vi "Sched select tube mask.vi"(9 "sched61-80mask":u32, 10 "sched31-60mask":u32, 11 "sched1-30mask":u32) -> (1 "Close":bool, 2 "Load":bool, 3 "selected sched":string)   [LabVIEW 2023]
uses:
  Sched select.ctl
panel:
  out "schd61-80array":bool[](array[boolean])
  out "schd31-60array":bool[](array[boolean])
  out "schd1-30array":bool[](array[boolean])
  in  "stop":bool
  in  "Schedules":T1
  out "SchedNames":string[](array[string])
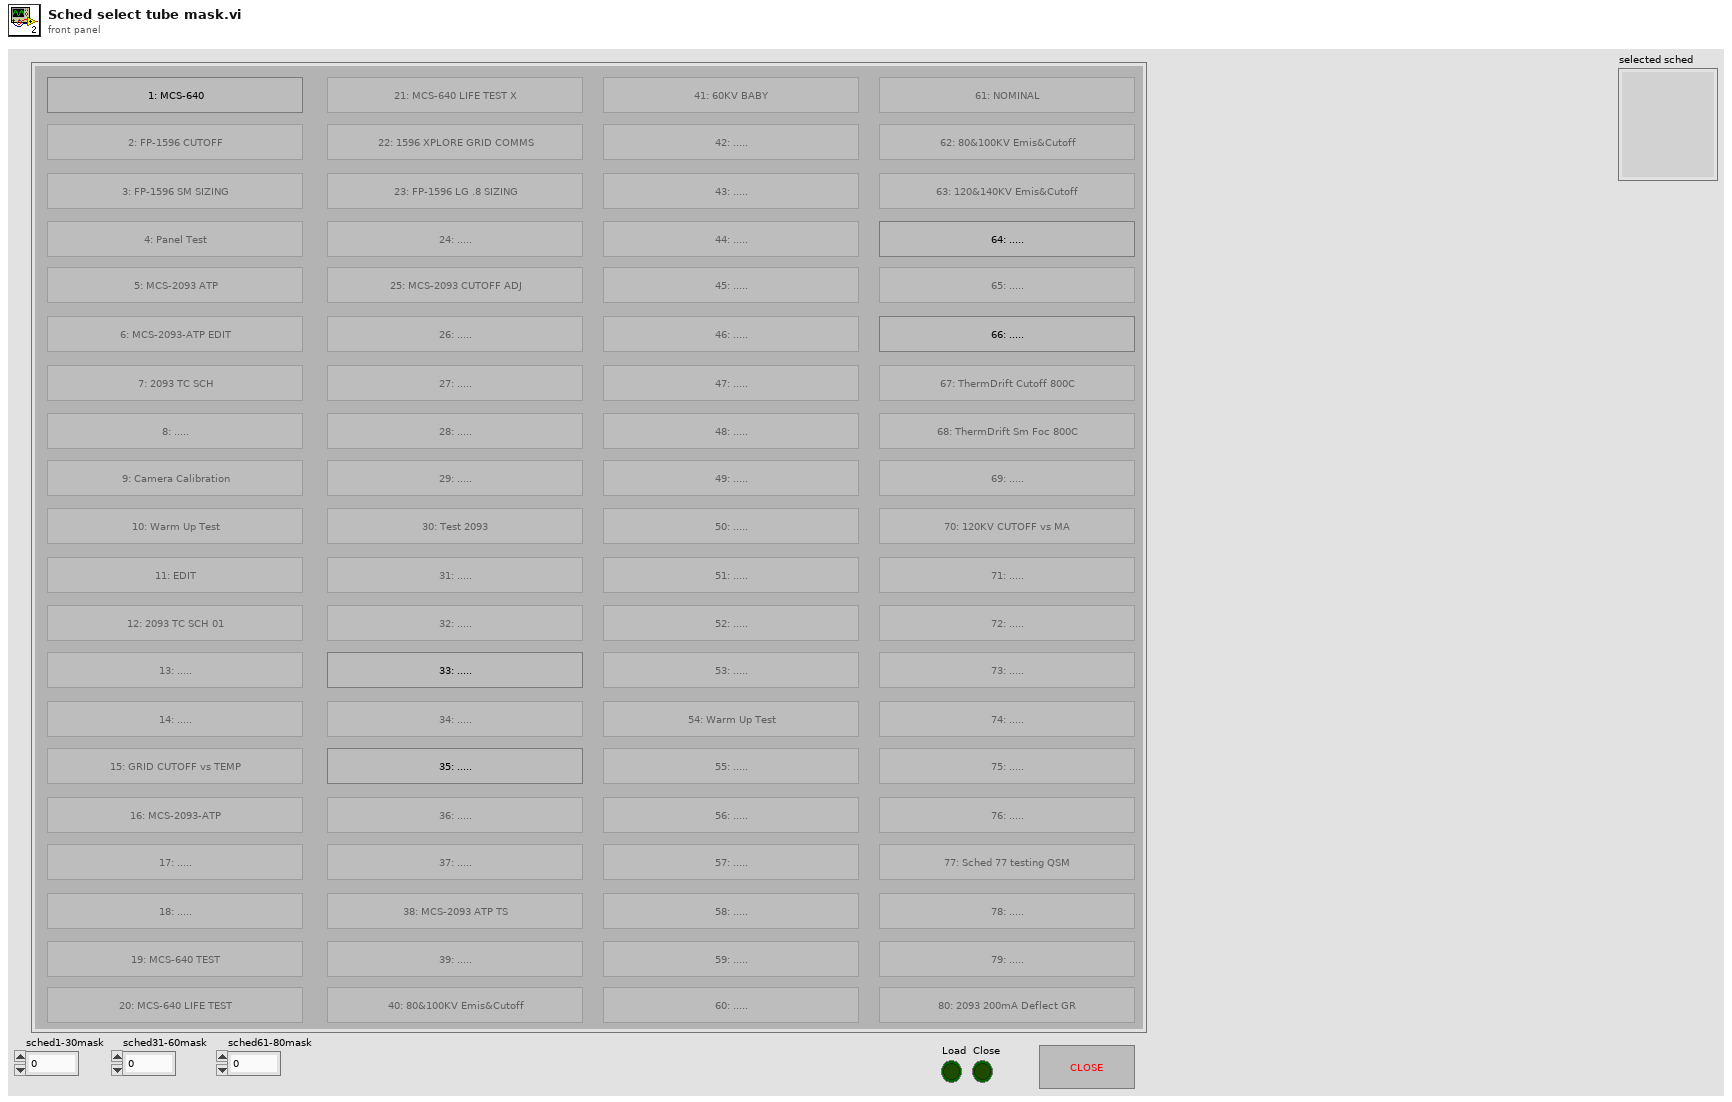
[diagram p1: front panel]
types:
  T1 = typedef "Sched select.ctl" = cluster{"OK Button 1":bool, "OK Button 2":bool, "OK Button 3":bool, "OK Button 4":bool, "OK Button 5":bool, "OK Button 6":bool, "OK Button 7":bool, "OK Button 8":bool, "OK Button 9":bool, "OK Button 10":bool, "OK Button 11":bool, "OK Button 12":bool, "OK Button 13":bool, "OK Button 14":bool, "OK Button 15":bool, "OK Button 16":bool, "OK Button 17":bool, "OK Button 18":bool, "OK Button 19":bool, "OK Button 20":bool, "OK Button 21":bool, "OK Button 22":bool, "OK Button 23":bool, "OK Button 24":bool, "OK Button 25":bool, "OK Button 26":bool, "OK Button 27":bool, "OK Button 28":bool, "OK Button 29":bool, "OK Button 30":bool, "OK Button 31":bool, "OK Button 32":bool, "OK Button 33":bool, "OK Button 34":bool, "OK Button 35":bool, "OK Button 36":bool, "OK Button 37":bool, "OK Button 38":bool, "OK Button 39":bool, "OK Button 40":bool, "OK Button 41":bool, "OK Button 42":bool, "OK Button 43":bool, "OK Button 44":bool, "OK Button 45":bool, "OK Button 46":bool, "OK Button 47":bool, "OK Button 48":bool, "OK Button 49":bool, "OK Button 50":bool, "OK Button 51":bool, "OK Button 52":bool, "OK Button 53":bool, "OK Button 54":bool, "OK Button 55":bool, "OK Button 56":bool, "OK Button 57":bool, "OK Button 58":bool, "OK Button 59":bool, "OK Button 60":bool, "OK Button 61":bool, "OK Button 62":bool, "OK Button 63":bool, "OK Button 64":bool, "OK Button 65":bool, "OK Button 66":bool, "OK Button 67":bool, "OK Button 68":bool, "OK Button 69":bool, "OK Button 70":bool, "OK Button 71":bool, "OK Button 72":bool, "OK Button 73":bool, "OK Button 74":bool, "OK Button 75":bool, "OK Button 76":bool, "OK Button 77":bool, "OK Button 78":bool, "OK Button 79":bool, "OK Button 80":bool}
  T2 = enum8{"Enabled", "Disabled", "Disabled and Grayed Out"}
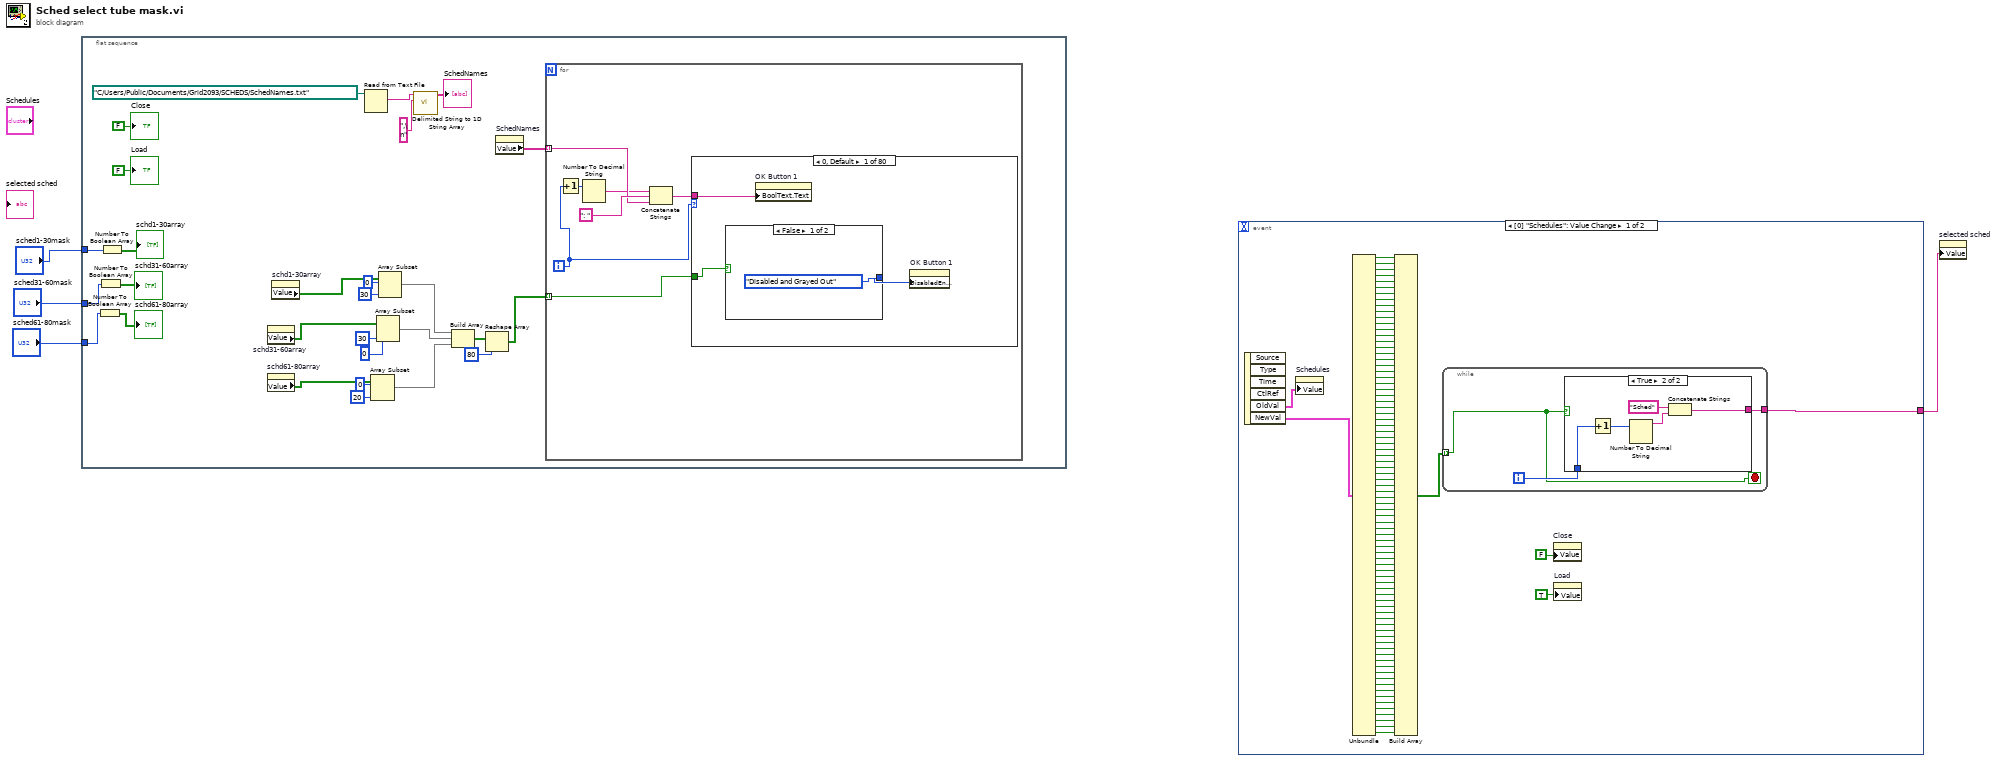
[diagram p0: block diagram]
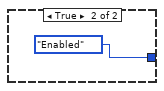
[diagram p2: hidden frame]
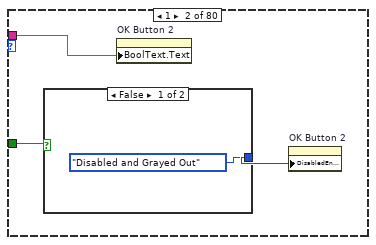
[diagram p3: hidden frame]
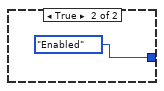
[diagram p4: hidden frame]
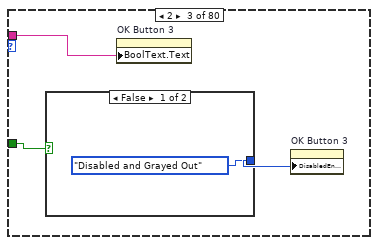
[diagram p5: hidden frame]
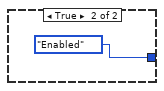
[diagram p6: hidden frame]
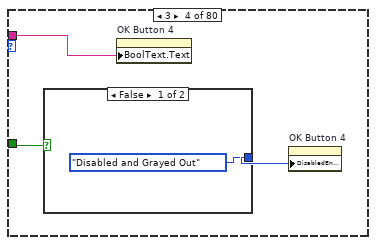
[diagram p7: hidden frame]
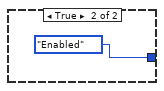
[diagram p8: hidden frame]
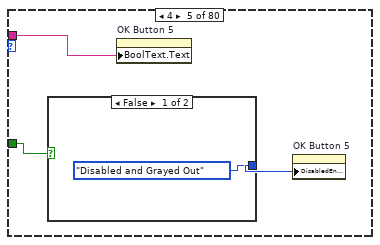
[diagram p9: hidden frame]
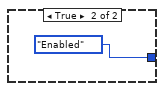
[diagram p10: hidden frame]
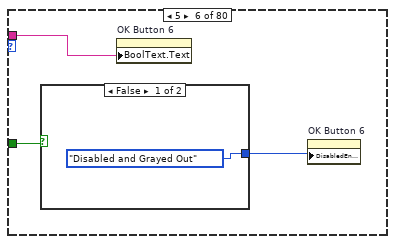
[diagram p11: hidden frame]
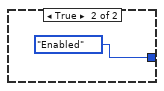
[diagram p12: hidden frame]
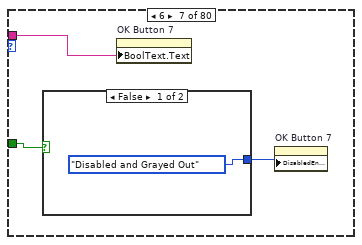
[diagram p13: hidden frame]
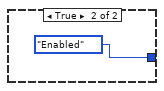
[diagram p14: hidden frame]
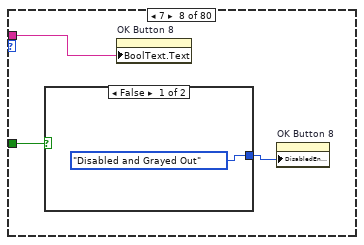
[diagram p15: hidden frame]
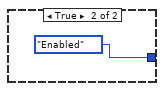
[diagram p16: hidden frame]
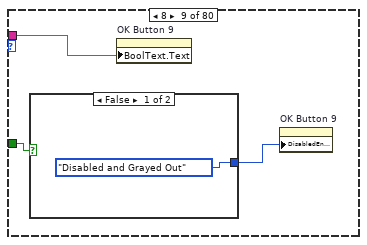
[diagram p17: hidden frame]
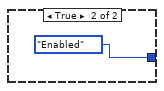
[diagram p18: hidden frame]
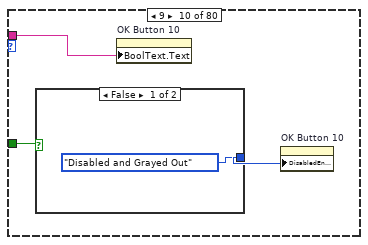
[diagram p19: hidden frame]
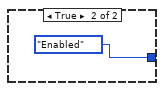
[diagram p20: hidden frame]
diagram:
  n1 = flat-sequence {
    tunnel: "sched1-30mask" -> [w22]
    tunnel: "sched31-60mask" -> [w21]
    tunnel: "sched61-80mask" -> [w20]
    frame #0 {
      n2 = Number To Boolean Array(number=w20) -> (Boolean array=→"schd61-80array":bool[])
      n3 = Number To Boolean Array(number=w21) -> (Boolean array=→"schd31-60array":bool[])
      n4 = Number To Boolean Array(number=w22) -> (Boolean array=→"schd1-30array":bool[])
      n5 = property on="schd31-60array" class="Arr (strict)"() -> ("Value"=w10:bool[])  [unwired: 2 in, 2 out]
      n6 = property on="schd61-80array" class="Arr (strict)"() -> ("Value"=w11:bool[])  [unwired: 2 in, 2 out]
      n7 = property on="schd1-30array" class="Arr (strict)"() -> ("Value"=w16:bool[])  [unwired: 2 in, 2 out]
      n8 = Read from Text File(file (use dialog)=path "C:/Users/Public/Documents/Grid2093/SCHEDS/SchedNames.txt") -> (text=w32:string)  [unwired: 3 in, 3 out]
      n9 = Array Subset(array=w11, index=0, length=20) -> (w9:bool[])
      n10 = Array Subset(array=w10, index=0, length=30) -> (w8:bool[])
      n11 = Array Subset(array=w16, index=0, length=30) -> (w14:bool[])
      n12 = call <vilib>:"Delimited String to 1D String Array.vi"("delimiter"=",\n", "delimited string"=w32) -> ("string array"=→"SchedNames":string[])  [unwired: 9 in]
      n13 = Build Array(w14, w8, w9) -> (w19:bool[][])
      n14 = Reshape Array(w19, 80 ("dimension size")) -> (w18:bool[])
      n15 = property on="SchedNames" class="Arr (strict)"() -> ("Value"=w29:string[])  [unwired: 2 in, 2 out]
      n16 = for {
        tunnel: w29 -> [w38] mode=indexing
        tunnel: w18 -> [w33] mode=indexing
        i -> [w35]
        n17 = Increment(x=w35) -> (x+1=w36:i32)
        n18 = Number To Decimal String(number=w36) -> (decimal integer string=w37:string)  [unwired: 1 in]
        n19 = Concatenate Strings(w37, ": " ("string"), w38) -> (w34:string)
        n20 = case shown="0, Default" w35 {
          tunnel: w34 -> [w42 w47 w52 w57 w62 w67 w72 w77 w82 w87 w92 w97 w102 w107 w112 w117 w122 w127 w132 w137 w142 w147 w152 w157 w162 w167 w172 w177 w182 w187 w192 w197 w202 w207 w212 w217 w222 w227 w232 w237 w242 w247 w252 w257 w262 w267 w272 w277 w282 w287 w292 w297 w302 w307 w312 w317 w322 w327 w332 w337 w342 w347 w352 w357 w362 w367 w372 w377 w382 w387 w392 w397 w402 w407 w412 w417 w422 w427 w432 w437]
          tunnel: w33 -> [w40 w45 w50 w55 w60 w65 w70 w75 w80 w85 w90 w95 w100 w105 w110 w115 w120 w125 w130 w135 w140 w145 w150 w155 w160 w165 w170 w175 w180 w185 w190 w195 w200 w205 w210 w215 w220 w225 w230 w235 w240 w245 w250 w255 w260 w265 w270 w275 w280 w285 w290 w295 w300 w305 w310 w315 w320 w325 w330 w335 w340 w345 w350 w355 w360 w365 w370 w375 w380 w385 w390 w395 w400 w405 w410 w415 w420 w425 w430 w435]
          frame 0, Default {
            n21 = case shown="False" w40 {
              tunnel: [T2."Disabled and Grayed Out" ("Disabled") T2."Enabled" ("Disabled")] -> w41
              frame False {
              }
              frame True {
              }
            }
            n22 = property on="OK Button 1" class="Bool (strict)"("BoolText.Text"=w42) -> ()  [unwired: 2 in, 2 out]
            n23 = property on="OK Button 1" class="Bool (strict)"("DisabledEnum"=w41) -> ()  [unwired: 2 in, 2 out]
          }
          frame 1 {
            n24 = case shown="False" w45 {
              tunnel: [T2."Disabled and Grayed Out" ("Disabled") T2."Enabled" ("Disabled")] -> w46
              frame False {
              }
              frame True {
              }
            }
            n25 = property on="OK Button 2" class="Bool (strict)"("BoolText.Text"=w47) -> ()  [unwired: 2 in, 2 out]
            n26 = property on="OK Button 2" class="Bool (strict)"("DisabledEnum"=w46) -> ()  [unwired: 2 in, 2 out]
          }
          frame 2 {
            n27 = case shown="False" w50 {
              tunnel: [T2."Disabled and Grayed Out" ("Disabled") T2."Enabled" ("Disabled")] -> w51
              frame False {
              }
              frame True {
              }
            }
            n28 = property on="OK Button 3" class="Bool (strict)"("BoolText.Text"=w52) -> ()  [unwired: 2 in, 2 out]
            n29 = property on="OK Button 3" class="Bool (strict)"("DisabledEnum"=w51) -> ()  [unwired: 2 in, 2 out]
          }
          frame 3 {
            n30 = case shown="False" w55 {
              tunnel: [T2."Disabled and Grayed Out" ("Disabled") T2."Enabled" ("Disabled")] -> w56
              frame False {
              }
              frame True {
              }
            }
            n31 = property on="OK Button 4" class="Bool (strict)"("BoolText.Text"=w57) -> ()  [unwired: 2 in, 2 out]
            n32 = property on="OK Button 4" class="Bool (strict)"("DisabledEnum"=w56) -> ()  [unwired: 2 in, 2 out]
          }
          frame 4 {
            n33 = case shown="False" w60 {
              tunnel: [T2."Disabled and Grayed Out" ("Disabled") T2."Enabled" ("Disabled")] -> w61
              frame False {
              }
              frame True {
              }
            }
            n34 = property on="OK Button 5" class="Bool (strict)"("BoolText.Text"=w62) -> ()  [unwired: 2 in, 2 out]
            n35 = property on="OK Button 5" class="Bool (strict)"("DisabledEnum"=w61) -> ()  [unwired: 2 in, 2 out]
          }
          frame 5 {
            n36 = case shown="False" w65 {
              tunnel: [T2."Disabled and Grayed Out" ("Disabled") T2."Enabled" ("Disabled")] -> w66
              frame False {
              }
              frame True {
              }
            }
            n37 = property on="OK Button 6" class="Bool (strict)"("BoolText.Text"=w67) -> ()  [unwired: 2 in, 2 out]
            n38 = property on="OK Button 6" class="Bool (strict)"("DisabledEnum"=w66) -> ()  [unwired: 2 in, 2 out]
          }
          frame 6 {
            n39 = case shown="False" w70 {
              tunnel: [T2."Disabled and Grayed Out" ("Disabled") T2."Enabled" ("Disabled")] -> w71
              frame False {
              }
              frame True {
              }
            }
            n40 = property on="OK Button 7" class="Bool (strict)"("BoolText.Text"=w72) -> ()  [unwired: 2 in, 2 out]
            n41 = property on="OK Button 7" class="Bool (strict)"("DisabledEnum"=w71) -> ()  [unwired: 2 in, 2 out]
          }
          frame 7 {
            n42 = case shown="False" w75 {
              tunnel: [T2."Disabled and Grayed Out" ("Disabled") T2."Enabled" ("Disabled")] -> w76
              frame False {
              }
              frame True {
              }
            }
            n43 = property on="OK Button 8" class="Bool (strict)"("BoolText.Text"=w77) -> ()  [unwired: 2 in, 2 out]
            n44 = property on="OK Button 8" class="Bool (strict)"("DisabledEnum"=w76) -> ()  [unwired: 2 in, 2 out]
          }
          frame 8 {
            n45 = case shown="False" w80 {
              tunnel: [T2."Disabled and Grayed Out" ("Disabled") T2."Enabled" ("Disabled")] -> w81
              frame False {
              }
              frame True {
              }
            }
            n46 = property on="OK Button 9" class="Bool (strict)"("BoolText.Text"=w82) -> ()  [unwired: 2 in, 2 out]
            n47 = property on="OK Button 9" class="Bool (strict)"("DisabledEnum"=w81) -> ()  [unwired: 2 in, 2 out]
          }
          frame 9 {
            n48 = case shown="False" w85 {
              tunnel: [T2."Disabled and Grayed Out" ("Disabled") T2."Enabled" ("Disabled")] -> w86
              frame False {
              }
              frame True {
              }
            }
            n49 = property on="OK Button 10" class="Bool (strict)"("BoolText.Text"=w87) -> ()  [unwired: 2 in, 2 out]
            n50 = property on="OK Button 10" class="Bool (strict)"("DisabledEnum"=w86) -> ()  [unwired: 2 in, 2 out]
          }
          frame 10 {
            n51 = case shown="False" w90 {
              tunnel: [T2."Disabled and Grayed Out" ("Disabled") T2."Enabled" ("Disabled")] -> w91
              frame False {
              }
              frame True {
              }
            }
            n52 = property on="OK Button 11" class="Bool (strict)"("BoolText.Text"=w92) -> ()  [unwired: 2 in, 2 out]
            n53 = property on="OK Button 11" class="Bool (strict)"("DisabledEnum"=w91) -> ()  [unwired: 2 in, 2 out]
          }
          frame 11 {
            n54 = case shown="False" w95 {
              tunnel: [T2."Disabled and Grayed Out" ("Disabled") T2."Enabled" ("Disabled")] -> w96
              frame False {
              }
              frame True {
              }
            }
            n55 = property on="OK Button 12" class="Bool (strict)"("BoolText.Text"=w97) -> ()  [unwired: 2 in, 2 out]
            n56 = property on="OK Button 12" class="Bool (strict)"("DisabledEnum"=w96) -> ()  [unwired: 2 in, 2 out]
          }
          frame 12 {
            n57 = case shown="False" w100 {
              tunnel: [T2."Disabled and Grayed Out" ("Disabled") T2."Enabled" ("Disabled")] -> w101
              frame False {
              }
              frame True {
              }
            }
            n58 = property on="OK Button 13" class="Bool (strict)"("BoolText.Text"=w102) -> ()  [unwired: 2 in, 2 out]
            n59 = property on="OK Button 13" class="Bool (strict)"("DisabledEnum"=w101) -> ()  [unwired: 2 in, 2 out]
          }
          frame 13 {
            n60 = case shown="False" w105 {
              tunnel: [T2."Disabled and Grayed Out" ("Disabled") T2."Enabled" ("Disabled")] -> w106
              frame False {
              }
              frame True {
              }
            }
            n61 = property on="OK Button 14" class="Bool (strict)"("BoolText.Text"=w107) -> ()  [unwired: 2 in, 2 out]
            n62 = property on="OK Button 14" class="Bool (strict)"("DisabledEnum"=w106) -> ()  [unwired: 2 in, 2 out]
          }
          frame 14 {
            n63 = case shown="False" w110 {
              tunnel: [T2."Disabled and Grayed Out" ("Disabled") T2."Enabled" ("Disabled")] -> w111
              frame False {
              }
              frame True {
              }
            }
            n64 = property on="OK Button 15" class="Bool (strict)"("BoolText.Text"=w112) -> ()  [unwired: 2 in, 2 out]
            n65 = property on="OK Button 15" class="Bool (strict)"("DisabledEnum"=w111) -> ()  [unwired: 2 in, 2 out]
          }
          frame 15 {
            n66 = case shown="False" w115 {
              tunnel: [T2."Disabled and Grayed Out" ("Disabled") T2."Enabled" ("Disabled")] -> w116
              frame False {
              }
              frame True {
              }
            }
            n67 = property on="OK Button 16" class="Bool (strict)"("BoolText.Text"=w117) -> ()  [unwired: 2 in, 2 out]
            n68 = property on="OK Button 16" class="Bool (strict)"("DisabledEnum"=w116) -> ()  [unwired: 2 in, 2 out]
          }
          frame 16 {
            n69 = case shown="False" w120 {
              tunnel: [T2."Disabled and Grayed Out" ("Disabled") T2."Enabled" ("Disabled")] -> w121
              frame False {
              }
              frame True {
              }
            }
            n70 = property on="OK Button 17" class="Bool (strict)"("BoolText.Text"=w122) -> ()  [unwired: 2 in, 2 out]
            n71 = property on="OK Button 17" class="Bool (strict)"("DisabledEnum"=w121) -> ()  [unwired: 2 in, 2 out]
          }
          frame 17 {
            n72 = case shown="False" w125 {
              tunnel: [T2."Disabled and Grayed Out" ("Disabled") T2."Enabled" ("Disabled")] -> w126
              frame False {
              }
              frame True {
              }
            }
            n73 = property on="OK Button 18" class="Bool (strict)"("BoolText.Text"=w127) -> ()  [unwired: 2 in, 2 out]
            n74 = property on="OK Button 18" class="Bool (strict)"("DisabledEnum"=w126) -> ()  [unwired: 2 in, 2 out]
          }
          frame 18 {
            n75 = case shown="False" w130 {
              tunnel: [T2."Disabled and Grayed Out" ("Disabled") T2."Enabled" ("Disabled")] -> w131
              frame False {
              }
              frame True {
              }
            }
            n76 = property on="OK Button 19" class="Bool (strict)"("BoolText.Text"=w132) -> ()  [unwired: 2 in, 2 out]
            n77 = property on="OK Button 19" class="Bool (strict)"("DisabledEnum"=w131) -> ()  [unwired: 2 in, 2 out]
          }
          frame 19 {
            n78 = case shown="False" w135 {
              tunnel: [T2."Disabled and Grayed Out" ("Disabled") T2."Enabled" ("Disabled")] -> w136
              frame False {
              }
              frame True {
              }
            }
            n79 = property on="OK Button 20" class="Bool (strict)"("BoolText.Text"=w137) -> ()  [unwired: 2 in, 2 out]
            n80 = property on="OK Button 20" class="Bool (strict)"("DisabledEnum"=w136) -> ()  [unwired: 2 in, 2 out]
          }
          frame 20 {
            n81 = case shown="False" w140 {
              tunnel: [T2."Disabled and Grayed Out" ("Disabled") T2."Enabled" ("Disabled")] -> w141
              frame False {
              }
              frame True {
              }
            }
            n82 = property on="OK Button 21" class="Bool (strict)"("BoolText.Text"=w142) -> ()  [unwired: 2 in, 2 out]
            n83 = property on="OK Button 21" class="Bool (strict)"("DisabledEnum"=w141) -> ()  [unwired: 2 in, 2 out]
          }
          frame 21 {
            n84 = case shown="False" w145 {
              tunnel: [T2."Disabled and Grayed Out" ("Disabled") T2."Enabled" ("Disabled")] -> w146
              frame False {
              }
              frame True {
              }
            }
            n85 = property on="OK Button 22" class="Bool (strict)"("BoolText.Text"=w147) -> ()  [unwired: 2 in, 2 out]
            n86 = property on="OK Button 22" class="Bool (strict)"("DisabledEnum"=w146) -> ()  [unwired: 2 in, 2 out]
          }
          frame 22 {
            n87 = case shown="False" w150 {
              tunnel: [T2."Disabled and Grayed Out" ("Disabled") T2."Enabled" ("Disabled")] -> w151
              frame False {
              }
              frame True {
              }
            }
            n88 = property on="OK Button 23" class="Bool (strict)"("BoolText.Text"=w152) -> ()  [unwired: 2 in, 2 out]
            n89 = property on="OK Button 23" class="Bool (strict)"("DisabledEnum"=w151) -> ()  [unwired: 2 in, 2 out]
          }
          frame 23 {
            n90 = case shown="False" w155 {
              tunnel: [T2."Disabled and Grayed Out" ("Disabled") T2."Enabled" ("Disabled")] -> w156
              frame False {
              }
              frame True {
              }
            }
            n91 = property on="OK Button 24" class="Bool (strict)"("BoolText.Text"=w157) -> ()  [unwired: 2 in, 2 out]
            n92 = property on="OK Button 24" class="Bool (strict)"("DisabledEnum"=w156) -> ()  [unwired: 2 in, 2 out]
          }
          frame 24 {
            n93 = case shown="False" w160 {
              tunnel: [T2."Disabled and Grayed Out" ("Disabled") T2."Enabled" ("Disabled")] -> w161
              frame False {
              }
              frame True {
              }
            }
            n94 = property on="OK Button 25" class="Bool (strict)"("BoolText.Text"=w162) -> ()  [unwired: 2 in, 2 out]
            n95 = property on="OK Button 25" class="Bool (strict)"("DisabledEnum"=w161) -> ()  [unwired: 2 in, 2 out]
          }
          frame 25 {
            n96 = case shown="False" w165 {
              tunnel: [T2."Disabled and Grayed Out" ("Disabled") T2."Enabled" ("Disabled")] -> w166
              frame False {
              }
              frame True {
              }
            }
            n97 = property on="OK Button 26" class="Bool (strict)"("BoolText.Text"=w167) -> ()  [unwired: 2 in, 2 out]
            n98 = property on="OK Button 26" class="Bool (strict)"("DisabledEnum"=w166) -> ()  [unwired: 2 in, 2 out]
          }
          frame 26 {
            n99 = case shown="False" w170 {
              tunnel: [T2."Disabled and Grayed Out" ("Disabled") T2."Enabled" ("Disabled")] -> w171
              frame False {
              }
              frame True {
              }
            }
            n100 = property on="OK Button 27" class="Bool (strict)"("BoolText.Text"=w172) -> ()  [unwired: 2 in, 2 out]
            n101 = property on="OK Button 27" class="Bool (strict)"("DisabledEnum"=w171) -> ()  [unwired: 2 in, 2 out]
          }
          frame 27 {
            n102 = case shown="False" w175 {
              tunnel: [T2."Disabled and Grayed Out" ("Disabled") T2."Enabled" ("Disabled")] -> w176
              frame False {
              }
              frame True {
              }
            }
            n103 = property on="OK Button 28" class="Bool (strict)"("BoolText.Text"=w177) -> ()  [unwired: 2 in, 2 out]
            n104 = property on="OK Button 28" class="Bool (strict)"("DisabledEnum"=w176) -> ()  [unwired: 2 in, 2 out]
          }
          frame 28 {
            n105 = case shown="False" w180 {
              tunnel: [T2."Disabled and Grayed Out" ("Disabled") T2."Enabled" ("Disabled")] -> w181
              frame False {
              }
              frame True {
              }
            }
            n106 = property on="OK Button 29" class="Bool (strict)"("BoolText.Text"=w182) -> ()  [unwired: 2 in, 2 out]
            n107 = property on="OK Button 29" class="Bool (strict)"("DisabledEnum"=w181) -> ()  [unwired: 2 in, 2 out]
          }
          frame 29 {
            n108 = case shown="False" w185 {
              tunnel: [T2."Disabled and Grayed Out" ("Disabled") T2."Enabled" ("Disabled")] -> w186
              frame False {
              }
              frame True {
              }
            }
            n109 = property on="OK Button 30" class="Bool (strict)"("BoolText.Text"=w187) -> ()  [unwired: 2 in, 2 out]
            n110 = property on="OK Button 30" class="Bool (strict)"("DisabledEnum"=w186) -> ()  [unwired: 2 in, 2 out]
          }
          frame 30 {
            n111 = case shown="False" w190 {
              tunnel: [T2."Disabled and Grayed Out" ("Disabled") T2."Enabled" ("Disabled")] -> w191
              frame False {
              }
              frame True {
              }
            }
            n112 = property on="OK Button 31" class="Bool (strict)"("BoolText.Text"=w192) -> ()  [unwired: 2 in, 2 out]
            n113 = property on="OK Button 31" class="Bool (strict)"("DisabledEnum"=w191) -> ()  [unwired: 2 in, 2 out]
          }
          frame 31 {
            n114 = case shown="False" w195 {
              tunnel: [T2."Disabled and Grayed Out" ("Disabled") T2."Enabled" ("Disabled")] -> w196
              frame False {
              }
              frame True {
              }
            }
            n115 = property on="OK Button 32" class="Bool (strict)"("BoolText.Text"=w197) -> ()  [unwired: 2 in, 2 out]
            n116 = property on="OK Button 32" class="Bool (strict)"("DisabledEnum"=w196) -> ()  [unwired: 2 in, 2 out]
          }
          frame 32 {
            n117 = case shown="False" w200 {
              tunnel: [T2."Disabled and Grayed Out" ("Disabled") T2."Enabled" ("Disabled")] -> w201
              frame False {
              }
              frame True {
              }
            }
            n118 = property on="OK Button 33" class="Bool (strict)"("BoolText.Text"=w202) -> ()  [unwired: 2 in, 2 out]
            n119 = property on="OK Button 33" class="Bool (strict)"("DisabledEnum"=w201) -> ()  [unwired: 2 in, 2 out]
          }
          frame 33 {
            n120 = case shown="False" w205 {
              tunnel: [T2."Disabled and Grayed Out" ("Disabled") T2."Enabled" ("Disabled")] -> w206
              frame False {
              }
              frame True {
              }
            }
            n121 = property on="OK Button 34" class="Bool (strict)"("BoolText.Text"=w207) -> ()  [unwired: 2 in, 2 out]
            n122 = property on="OK Button 34" class="Bool (strict)"("DisabledEnum"=w206) -> ()  [unwired: 2 in, 2 out]
          }
          frame 34 {
            n123 = case shown="False" w210 {
              tunnel: [T2."Disabled and Grayed Out" ("Disabled") T2."Enabled" ("Disabled")] -> w211
              frame False {
              }
              frame True {
              }
            }
            n124 = property on="OK Button 35" class="Bool (strict)"("BoolText.Text"=w212) -> ()  [unwired: 2 in, 2 out]
            n125 = property on="OK Button 35" class="Bool (strict)"("DisabledEnum"=w211) -> ()  [unwired: 2 in, 2 out]
          }
          frame 35 {
            n126 = case shown="False" w215 {
              tunnel: [T2."Disabled and Grayed Out" ("Disabled") T2."Enabled" ("Disabled")] -> w216
              frame False {
              }
              frame True {
              }
            }
            n127 = property on="OK Button 36" class="Bool (strict)"("BoolText.Text"=w217) -> ()  [unwired: 2 in, 2 out]
            n128 = property on="OK Button 36" class="Bool (strict)"("DisabledEnum"=w216) -> ()  [unwired: 2 in, 2 out]
          }
          frame 36 {
            n129 = case shown="False" w220 {
              tunnel: [T2."Disabled and Grayed Out" ("Disabled") T2."Enabled" ("Disabled")] -> w221
              frame False {
              }
              frame True {
              }
            }
            n130 = property on="OK Button 37" class="Bool (strict)"("BoolText.Text"=w222) -> ()  [unwired: 2 in, 2 out]
            n131 = property on="OK Button 37" class="Bool (strict)"("DisabledEnum"=w221) -> ()  [unwired: 2 in, 2 out]
          }
          frame 37 {
            n132 = case shown="False" w225 {
              tunnel: [T2."Disabled and Grayed Out" ("Disabled") T2."Enabled" ("Disabled")] -> w226
              frame False {
              }
              frame True {
              }
            }
            n133 = property on="OK Button 38" class="Bool (strict)"("BoolText.Text"=w227) -> ()  [unwired: 2 in, 2 out]
            n134 = property on="OK Button 38" class="Bool (strict)"("DisabledEnum"=w226) -> ()  [unwired: 2 in, 2 out]
          }
          frame 38 {
            n135 = case shown="False" w230 {
              tunnel: [T2."Disabled and Grayed Out" ("Disabled") T2."Enabled" ("Disabled")] -> w231
              frame False {
              }
              frame True {
              }
            }
            n136 = property on="OK Button 39" class="Bool (strict)"("BoolText.Text"=w232) -> ()  [unwired: 2 in, 2 out]
            n137 = property on="OK Button 39" class="Bool (strict)"("DisabledEnum"=w231) -> ()  [unwired: 2 in, 2 out]
          }
          frame 39 {
            n138 = case shown="False" w235 {
              tunnel: [T2."Disabled and Grayed Out" ("Disabled") T2."Enabled" ("Disabled")] -> w236
              frame False {
              }
              frame True {
              }
            }
            n139 = property on="OK Button 40" class="Bool (strict)"("BoolText.Text"=w237) -> ()  [unwired: 2 in, 2 out]
            n140 = property on="OK Button 40" class="Bool (strict)"("DisabledEnum"=w236) -> ()  [unwired: 2 in, 2 out]
          }
          frame 40 {
            n141 = case shown="False" w240 {
              tunnel: [T2."Disabled and Grayed Out" ("Disabled") T2."Enabled" ("Disabled")] -> w241
              frame False {
              }
              frame True {
              }
            }
            n142 = property on="OK Button 41" class="Bool (strict)"("BoolText.Text"=w242) -> ()  [unwired: 2 in, 2 out]
            n143 = property on="OK Button 41" class="Bool (strict)"("DisabledEnum"=w241) -> ()  [unwired: 2 in, 2 out]
          }
          frame 41 {
            n144 = case shown="False" w245 {
              tunnel: [T2."Disabled and Grayed Out" ("Disabled") T2."Enabled" ("Disabled")] -> w246
              frame False {
              }
              frame True {
              }
            }
            n145 = property on="OK Button 42" class="Bool (strict)"("BoolText.Text"=w247) -> ()  [unwired: 2 in, 2 out]
            n146 = property on="OK Button 42" class="Bool (strict)"("DisabledEnum"=w246) -> ()  [unwired: 2 in, 2 out]
          }
          frame 42 {
            n147 = case shown="False" w250 {
              tunnel: [T2."Disabled and Grayed Out" ("Disabled") T2."Enabled" ("Disabled")] -> w251
              frame False {
              }
              frame True {
              }
            }
            n148 = property on="OK Button 43" class="Bool (strict)"("BoolText.Text"=w252) -> ()  [unwired: 2 in, 2 out]
            n149 = property on="OK Button 43" class="Bool (strict)"("DisabledEnum"=w251) -> ()  [unwired: 2 in, 2 out]
          }
          frame 43 {
            n150 = case shown="False" w255 {
              tunnel: [T2."Disabled and Grayed Out" ("Disabled") T2."Enabled" ("Disabled")] -> w256
              frame False {
              }
              frame True {
              }
            }
            n151 = property on="OK Button 44" class="Bool (strict)"("BoolText.Text"=w257) -> ()  [unwired: 2 in, 2 out]
            n152 = property on="OK Button 44" class="Bool (strict)"("DisabledEnum"=w256) -> ()  [unwired: 2 in, 2 out]
          }
          frame 44 {
            n153 = case shown="False" w260 {
              tunnel: [T2."Disabled and Grayed Out" ("Disabled") T2."Enabled" ("Disabled")] -> w261
              frame False {
              }
              frame True {
              }
            }
            n154 = property on="OK Button 45" class="Bool (strict)"("BoolText.Text"=w262) -> ()  [unwired: 2 in, 2 out]
            n155 = property on="OK Button 45" class="Bool (strict)"("DisabledEnum"=w261) -> ()  [unwired: 2 in, 2 out]
          }
          frame 45 {
            n156 = case shown="False" w265 {
              tunnel: [T2."Disabled and Grayed Out" ("Disabled") T2."Enabled" ("Disabled")] -> w266
              frame False {
              }
              frame True {
              }
            }
            n157 = property on="OK Button 46" class="Bool (strict)"("BoolText.Text"=w267) -> ()  [unwired: 2 in, 2 out]
            n158 = property on="OK Button 46" class="Bool (strict)"("DisabledEnum"=w266) -> ()  [unwired: 2 in, 2 out]
          }
          frame 46 {
            n159 = case shown="False" w270 {
              tunnel: [T2."Disabled and Grayed Out" ("Disabled") T2."Enabled" ("Disabled")] -> w271
              frame False {
              }
              frame True {
              }
            }
            n160 = property on="OK Button 47" class="Bool (strict)"("BoolText.Text"=w272) -> ()  [unwired: 2 in, 2 out]
            n161 = property on="OK Button 47" class="Bool (strict)"("DisabledEnum"=w271) -> ()  [unwired: 2 in, 2 out]
          }
          frame 47 {
            n162 = case shown="False" w275 {
              tunnel: [T2."Disabled and Grayed Out" ("Disabled") T2."Enabled" ("Disabled")] -> w276
              frame False {
              }
              frame True {
              }
            }
            n163 = property on="OK Button 48" class="Bool (strict)"("BoolText.Text"=w277) -> ()  [unwired: 2 in, 2 out]
            n164 = property on="OK Button 48" class="Bool (strict)"("DisabledEnum"=w276) -> ()  [unwired: 2 in, 2 out]
          }
          frame 48 {
            n165 = case shown="False" w280 {
              tunnel: [T2."Disabled and Grayed Out" ("Disabled") T2."Enabled" ("Disabled")] -> w281
              frame False {
              }
              frame True {
              }
            }
            n166 = property on="OK Button 49" class="Bool (strict)"("BoolText.Text"=w282) -> ()  [unwired: 2 in, 2 out]
            n167 = property on="OK Button 49" class="Bool (strict)"("DisabledEnum"=w281) -> ()  [unwired: 2 in, 2 out]
          }
          frame 49 {
            n168 = case shown="False" w285 {
              tunnel: [T2."Disabled and Grayed Out" ("Disabled") T2."Enabled" ("Disabled")] -> w286
              frame False {
              }
              frame True {
              }
            }
            n169 = property on="OK Button 50" class="Bool (strict)"("BoolText.Text"=w287) -> ()  [unwired: 2 in, 2 out]
            n170 = property on="OK Button 50" class="Bool (strict)"("DisabledEnum"=w286) -> ()  [unwired: 2 in, 2 out]
          }
          frame 50 {
            n171 = case shown="False" w290 {
              tunnel: [T2."Disabled and Grayed Out" ("Disabled") T2."Enabled" ("Disabled")] -> w291
              frame False {
              }
              frame True {
              }
            }
            n172 = property on="OK Button 51" class="Bool (strict)"("BoolText.Text"=w292) -> ()  [unwired: 2 in, 2 out]
            n173 = property on="OK Button 51" class="Bool (strict)"("DisabledEnum"=w291) -> ()  [unwired: 2 in, 2 out]
          }
          frame 51 {
            n174 = case shown="False" w295 {
              tunnel: [T2."Disabled and Grayed Out" ("Disabled") T2."Enabled" ("Disabled")] -> w296
              frame False {
              }
              frame True {
              }
            }
            n175 = property on="OK Button 52" class="Bool (strict)"("BoolText.Text"=w297) -> ()  [unwired: 2 in, 2 out]
            n176 = property on="OK Button 52" class="Bool (strict)"("DisabledEnum"=w296) -> ()  [unwired: 2 in, 2 out]
          }
          frame 52 {
            n177 = case shown="False" w300 {
              tunnel: [T2."Disabled and Grayed Out" ("Disabled") T2."Enabled" ("Disabled")] -> w301
              frame False {
              }
              frame True {
              }
            }
            n178 = property on="OK Button 53" class="Bool (strict)"("BoolText.Text"=w302) -> ()  [unwired: 2 in, 2 out]
            n179 = property on="OK Button 53" class="Bool (strict)"("DisabledEnum"=w301) -> ()  [unwired: 2 in, 2 out]
          }
          frame 53 {
            n180 = case shown="False" w305 {
              tunnel: [T2."Disabled and Grayed Out" ("Disabled") T2."Enabled" ("Disabled")] -> w306
              frame False {
              }
              frame True {
              }
            }
            n181 = property on="OK Button 54" class="Bool (strict)"("BoolText.Text"=w307) -> ()  [unwired: 2 in, 2 out]
            n182 = property on="OK Button 54" class="Bool (strict)"("DisabledEnum"=w306) -> ()  [unwired: 2 in, 2 out]
          }
          frame 54 {
            n183 = case shown="False" w310 {
              tunnel: [T2."Disabled and Grayed Out" ("Disabled") T2."Enabled" ("Disabled")] -> w311
              frame False {
              }
              frame True {
              }
            }
            n184 = property on="OK Button 55" class="Bool (strict)"("BoolText.Text"=w312) -> ()  [unwired: 2 in, 2 out]
            n185 = property on="OK Button 55" class="Bool (strict)"("DisabledEnum"=w311) -> ()  [unwired: 2 in, 2 out]
          }
          frame 55 {
            n186 = case shown="False" w315 {
              tunnel: [T2."Disabled and Grayed Out" ("Disabled") T2."Enabled" ("Disabled")] -> w316
              frame False {
              }
              frame True {
              }
            }
            n187 = property on="OK Button 56" class="Bool (strict)"("BoolText.Text"=w317) -> ()  [unwired: 2 in, 2 out]
            n188 = property on="OK Button 56" class="Bool (strict)"("DisabledEnum"=w316) -> ()  [unwired: 2 in, 2 out]
          }
          frame 56 {
            n189 = case shown="False" w320 {
              tunnel: [T2."Disabled and Grayed Out" ("Disabled") T2."Enabled" ("Disabled")] -> w321
              frame False {
              }
              frame True {
              }
            }
            n190 = property on="OK Button 57" class="Bool (strict)"("BoolText.Text"=w322) -> ()  [unwired: 2 in, 2 out]
            n191 = property on="OK Button 57" class="Bool (strict)"("DisabledEnum"=w321) -> ()  [unwired: 2 in, 2 out]
          }
          frame 57 {
            n192 = case shown="False" w325 {
              tunnel: [T2."Disabled and Grayed Out" ("Disabled") T2."Enabled" ("Disabled")] -> w326
              frame False {
              }
              frame True {
              }
            }
            n193 = property on="OK Button 58" class="Bool (strict)"("BoolText.Text"=w327) -> ()  [unwired: 2 in, 2 out]
            n194 = property on="OK Button 58" class="Bool (strict)"("DisabledEnum"=w326) -> ()  [unwired: 2 in, 2 out]
          }
          frame 58 {
            n195 = case shown="False" w330 {
              tunnel: [T2."Disabled and Grayed Out" ("Disabled") T2."Enabled" ("Disabled")] -> w331
              frame False {
              }
              frame True {
              }
            }
            n196 = property on="OK Button 59" class="Bool (strict)"("BoolText.Text"=w332) -> ()  [unwired: 2 in, 2 out]
            n197 = property on="OK Button 59" class="Bool (strict)"("DisabledEnum"=w331) -> ()  [unwired: 2 in, 2 out]
          }
          frame 59 {
            n198 = case shown="False" w335 {
              tunnel: [T2."Disabled and Grayed Out" ("Disabled") T2."Enabled" ("Disabled")] -> w336
              frame False {
              }
              frame True {
              }
            }
            n199 = property on="OK Button 60" class="Bool (strict)"("BoolText.Text"=w337) -> ()  [unwired: 2 in, 2 out]
            n200 = property on="OK Button 60" class="Bool (strict)"("DisabledEnum"=w336) -> ()  [unwired: 2 in, 2 out]
          }
          frame 60 {
            n201 = case shown="False" w340 {
              tunnel: [T2."Disabled and Grayed Out" ("Disabled") T2."Enabled" ("Disabled")] -> w341
              frame False {
              }
              frame True {
              }
            }
            n202 = property on="OK Button 61" class="Bool (strict)"("BoolText.Text"=w342) -> ()  [unwired: 2 in, 2 out]
            n203 = property on="OK Button 61" class="Bool (strict)"("DisabledEnum"=w341) -> ()  [unwired: 2 in, 2 out]
          }
          frame 61 {
            n204 = case shown="False" w345 {
              tunnel: [T2."Disabled and Grayed Out" ("Disabled") T2."Enabled" ("Disabled")] -> w346
              frame False {
              }
              frame True {
              }
            }
            n205 = property on="OK Button 62" class="Bool (strict)"("BoolText.Text"=w347) -> ()  [unwired: 2 in, 2 out]
            n206 = property on="OK Button 62" class="Bool (strict)"("DisabledEnum"=w346) -> ()  [unwired: 2 in, 2 out]
          }
          frame 62 {
            n207 = case shown="False" w350 {
              tunnel: [T2."Disabled and Grayed Out" ("Disabled") T2."Enabled" ("Disabled")] -> w351
              frame False {
              }
              frame True {
              }
            }
            n208 = property on="OK Button 63" class="Bool (strict)"("BoolText.Text"=w352) -> ()  [unwired: 2 in, 2 out]
            n209 = property on="OK Button 63" class="Bool (strict)"("DisabledEnum"=w351) -> ()  [unwired: 2 in, 2 out]
          }
          frame 63 {
            n210 = case shown="False" w355 {
              tunnel: [T2."Disabled and Grayed Out" ("Disabled") T2."Enabled" ("Disabled")] -> w356
              frame False {
              }
              frame True {
              }
            }
            n211 = property on="OK Button 64" class="Bool (strict)"("BoolText.Text"=w357) -> ()  [unwired: 2 in, 2 out]
            n212 = property on="OK Button 64" class="Bool (strict)"("DisabledEnum"=w356) -> ()  [unwired: 2 in, 2 out]
          }
          frame 64 {
            n213 = case shown="False" w360 {
              tunnel: [T2."Disabled and Grayed Out" ("Disabled") T2."Enabled" ("Disabled")] -> w361
              frame False {
              }
              frame True {
              }
            }
            n214 = property on="OK Button 65" class="Bool (strict)"("BoolText.Text"=w362) -> ()  [unwired: 2 in, 2 out]
            n215 = property on="OK Button 65" class="Bool (strict)"("DisabledEnum"=w361) -> ()  [unwired: 2 in, 2 out]
          }
          frame 65 {
            n216 = case shown="False" w365 {
              tunnel: [T2."Disabled and Grayed Out" ("Disabled") T2."Enabled" ("Disabled")] -> w366
              frame False {
              }
              frame True {
              }
            }
            n217 = property on="OK Button 66" class="Bool (strict)"("BoolText.Text"=w367) -> ()  [unwired: 2 in, 2 out]
            n218 = property on="OK Button 66" class="Bool (strict)"("DisabledEnum"=w366) -> ()  [unwired: 2 in, 2 out]
          }
          frame 66 {
            n219 = case shown="False" w370 {
              tunnel: [T2."Disabled and Grayed Out" ("Disabled") T2."Enabled" ("Disabled")] -> w371
              frame False {
              }
              frame True {
              }
            }
            n220 = property on="OK Button 67" class="Bool (strict)"("BoolText.Text"=w372) -> ()  [unwired: 2 in, 2 out]
            n221 = property on="OK Button 67" class="Bool (strict)"("DisabledEnum"=w371) -> ()  [unwired: 2 in, 2 out]
          }
          frame 67 {
            n222 = case shown="False" w375 {
              tunnel: [T2."Disabled and Grayed Out" ("Disabled") T2."Enabled" ("Disabled")] -> w376
              frame False {
              }
              frame True {
              }
            }
            n223 = property on="OK Button 68" class="Bool (strict)"("BoolText.Text"=w377) -> ()  [unwired: 2 in, 2 out]
            n224 = property on="OK Button 68" class="Bool (strict)"("DisabledEnum"=w376) -> ()  [unwired: 2 in, 2 out]
          }
          frame 68 {
            n225 = case shown="False" w380 {
              tunnel: [T2."Disabled and Grayed Out" ("Disabled") T2."Enabled" ("Disabled")] -> w381
              frame False {
              }
              frame True {
              }
            }
            n226 = property on="OK Button 69" class="Bool (strict)"("BoolText.Text"=w382) -> ()  [unwired: 2 in, 2 out]
            n227 = property on="OK Button 69" class="Bool (strict)"("DisabledEnum"=w381) -> ()  [unwired: 2 in, 2 out]
          }
          frame 69 {
            n228 = case shown="False" w385 {
              tunnel: [T2."Disabled and Grayed Out" ("Disabled") T2."Enabled" ("Disabled")] -> w386
              frame False {
              }
              frame True {
              }
            }
            n229 = property on="OK Button 70" class="Bool (strict)"("BoolText.Text"=w387) -> ()  [unwired: 2 in, 2 out]
            n230 = property on="OK Button 70" class="Bool (strict)"("DisabledEnum"=w386) -> ()  [unwired: 2 in, 2 out]
          }
          frame 70 {
            n231 = case shown="False" w390 {
              tunnel: [T2."Disabled and Grayed Out" ("Disabled") T2."Enabled" ("Disabled")] -> w391
              frame False {
              }
              frame True {
              }
            }
            n232 = property on="OK Button 71" class="Bool (strict)"("BoolText.Text"=w392) -> ()  [unwired: 2 in, 2 out]
            n233 = property on="OK Button 71" class="Bool (strict)"("DisabledEnum"=w391) -> ()  [unwired: 2 in, 2 out]
          }
          frame 71 {
            n234 = case shown="False" w395 {
              tunnel: [T2."Disabled and Grayed Out" ("Disabled") T2."Enabled" ("Disabled")] -> w396
              frame False {
              }
              frame True {
              }
            }
            n235 = property on="OK Button 72" class="Bool (strict)"("BoolText.Text"=w397) -> ()  [unwired: 2 in, 2 out]
            n236 = property on="OK Button 72" class="Bool (strict)"("DisabledEnum"=w396) -> ()  [unwired: 2 in, 2 out]
          }
          frame 72 {
            n237 = case shown="False" w400 {
              tunnel: [T2."Disabled and Grayed Out" ("Disabled") T2."Enabled" ("Disabled")] -> w401
              frame False {
              }
              frame True {
              }
            }
            n238 = property on="OK Button 73" class="Bool (strict)"("BoolText.Text"=w402) -> ()  [unwired: 2 in, 2 out]
            n239 = property on="OK Button 73" class="Bool (strict)"("DisabledEnum"=w401) -> ()  [unwired: 2 in, 2 out]
          }
          frame 73 {
            n240 = case shown="False" w405 {
              tunnel: [T2."Disabled and Grayed Out" ("Disabled") T2."Enabled" ("Disabled")] -> w406
              frame False {
              }
              frame True {
              }
            }
            n241 = property on="OK Button 74" class="Bool (strict)"("BoolText.Text"=w407) -> ()  [unwired: 2 in, 2 out]
            n242 = property on="OK Button 74" class="Bool (strict)"("DisabledEnum"=w406) -> ()  [unwired: 2 in, 2 out]
          }
          frame 74 {
            n243 = case shown="False" w410 {
              tunnel: [T2."Disabled and Grayed Out" ("Disabled") T2."Enabled" ("Disabled")] -> w411
              frame False {
              }
              frame True {
              }
            }
            n244 = property on="OK Button 75" class="Bool (strict)"("BoolText.Text"=w412) -> ()  [unwired: 2 in, 2 out]
            n245 = property on="OK Button 75" class="Bool (strict)"("DisabledEnum"=w411) -> ()  [unwired: 2 in, 2 out]
          }
          frame 75 {
            n246 = case shown="False" w415 {
              tunnel: [T2."Disabled and Grayed Out" ("Disabled") T2."Enabled" ("Disabled")] -> w416
              frame False {
              }
              frame True {
              }
            }
            n247 = property on="OK Button 76" class="Bool (strict)"("BoolText.Text"=w417) -> ()  [unwired: 2 in, 2 out]
            n248 = property on="OK Button 76" class="Bool (strict)"("DisabledEnum"=w416) -> ()  [unwired: 2 in, 2 out]
          }
          frame 76 {
            n249 = case shown="False" w420 {
              tunnel: [T2."Disabled and Grayed Out" ("Disabled") T2."Enabled" ("Disabled")] -> w421
              frame False {
              }
              frame True {
              }
            }
            n250 = property on="OK Button 77" class="Bool (strict)"("BoolText.Text"=w422) -> ()  [unwired: 2 in, 2 out]
            n251 = property on="OK Button 77" class="Bool (strict)"("DisabledEnum"=w421) -> ()  [unwired: 2 in, 2 out]
          }
          frame 77 {
            n252 = case shown="True" w425 {
              tunnel: [T2."Disabled and Grayed Out" ("Disabled") T2."Enabled" ("Disabled")] -> w426
              frame False {
              }
              frame True {
              }
            }
            n253 = property on="OK Button 78" class="Bool (strict)"("BoolText.Text"=w427) -> ()  [unwired: 2 in, 2 out]
            n254 = property on="OK Button 78" class="Bool (strict)"("DisabledEnum"=w426) -> ()  [unwired: 2 in, 2 out]
          }
          frame 78 {
            n255 = case shown="False" w430 {
              tunnel: [T2."Disabled and Grayed Out" ("Disabled") T2."Enabled" ("Disabled")] -> w431
              frame False {
              }
              frame True {
              }
            }
            n256 = property on="OK Button 79" class="Bool (strict)"("BoolText.Text"=w432) -> ()  [unwired: 2 in, 2 out]
            n257 = property on="OK Button 79" class="Bool (strict)"("DisabledEnum"=w431) -> ()  [unwired: 2 in, 2 out]
          }
          frame 79 {
            n258 = case shown="False" w435 {
              tunnel: [T2."Disabled and Grayed Out" ("Disabled") T2."Enabled" ("Disabled")] -> w436
              frame False {
              }
              frame True {
              }
            }
            n259 = property on="OK Button 80" class="Bool (strict)"("BoolText.Text"=w437) -> ()  [unwired: 2 in, 2 out]
            n260 = property on="OK Button 80" class="Bool (strict)"("DisabledEnum"=w436) -> ()  [unwired: 2 in, 2 out]
          }
        }
      }
      "Close" <- FALSE ("Close")
      "Load" <- FALSE ("Load")
    }
  }
  n261 = event shown="[0] \"Schedules\": Value Change" {
    selector: _ -> [_ _]
    dyn-events: _ -> [_ _]
    timeout: _ -> [_ _]
    tunnel: [w444 _] -> w4
    event Value Change {
      n262 = event-data() -> ("OldVal"=w440:T1, "NewVal"=w441:T1)  [unwired: 1 in, 4 out]
      n263 = property on="Schedules" class="Clust (strict)"("Value"=w440) -> ()  [unwired: 2 in, 2 out]
      n264 = Unbundle(w441) -> ("OK Button 1"=w446:bool, "OK Button 2"=w447:bool, "OK Button 3"=w448:bool, "OK Button 4"=w449:bool, "OK Button 5"=w450:bool, "OK Button 6"=w451:bool, "OK Button 7"=w452:bool, "OK Button 8"=w453:bool, "OK Button 9"=w454:bool, "OK Button 10"=w455:bool, "OK Button 11"=w456:bool, "OK Button 12"=w457:bool, "OK Button 13"=w458:bool, "OK Button 14"=w459:bool, "OK Button 15"=w460:bool, "OK Button 16"=w461:bool, "OK Button 17"=w462:bool, "OK Button 18"=w463:bool, "OK Button 19"=w464:bool, "OK Button 20"=w465:bool, "OK Button 21"=w466:bool, "OK Button 22"=w467:bool, "OK Button 23"=w468:bool, "OK Button 24"=w469:bool, "OK Button 25"=w470:bool, "OK Button 26"=w471:bool, "OK Button 27"=w472:bool, "OK Button 28"=w473:bool, "OK Button 29"=w474:bool, "OK Button 30"=w475:bool, "OK Button 31"=w476:bool, "OK Button 32"=w477:bool, "OK Button 33"=w478:bool, "OK Button 34"=w479:bool, "OK Button 35"=w480:bool, "OK Button 36"=w481:bool, "OK Button 37"=w482:bool, "OK Button 38"=w483:bool, "OK Button 39"=w484:bool, "OK Button 40"=w485:bool, "OK Button 41"=w486:bool, "OK Button 42"=w487:bool, "OK Button 43"=w488:bool, "OK Button 44"=w489:bool, "OK Button 45"=w490:bool, "OK Button 46"=w491:bool, "OK Button 47"=w492:bool, "OK Button 48"=w493:bool, "OK Button 49"=w494:bool, "OK Button 50"=w495:bool, "OK Button 51"=w496:bool, "OK Button 52"=w497:bool, "OK Button 53"=w498:bool, "OK Button 54"=w499:bool, "OK Button 55"=w500:bool, "OK Button 56"=w501:bool, "OK Button 57"=w502:bool, "OK Button 58"=w503:bool, "OK Button 59"=w504:bool, "OK Button 60"=w505:bool, "OK Button 61"=w506:bool, "OK Button 62"=w507:bool, "OK Button 63"=w508:bool, "OK Button 64"=w509:bool, "OK Button 65"=w510:bool, "OK Button 66"=w511:bool, "OK Button 67"=w512:bool, "OK Button 68"=w513:bool, "OK Button 69"=w514:bool, "OK Button 70"=w516:bool, "OK Button 71"=w515:bool, "OK Button 72"=w517:bool, "OK Button 73"=w519:bool, "OK Button 74"=w518:bool, "OK Button 75"=w520:bool, "OK Button 76"=w521:bool, "OK Button 77"=w522:bool, "OK Button 78"=w523:bool, "OK Button 79"=w524:bool, "OK Button 80"=w525:bool)
      n265 = Build Array(w446, w447, w448, w449, w450, w451, w452, w453, w454, w455, w456, w457, w458, w459, w460, w461, w462, w463, w464, w465, w466, w467, w468, w469, w470, w471, w472, w473, w474, w475, w476, w477, w478, w479, w480, w481, w482, w483, w484, w485, w486, w487, w488, w489, w490, w491, w492, w493, w494, w495, w496, w497, w498, w499, w500, w501, w502, w503, w504, w505, w506, w507, w508, w509, w510, w511, w512, w513, w514, w516, w515, w517, w519, w518, w520, w521, w522, w523, w524, w525) -> (w445:bool[])
      n266 = while {
        tunnel: w445 -> [w526] mode=indexing
        tunnel: [w527] -> w444
        i -> [w528]
        stop <- w526 stop-if-true
        n267 = case shown="True" w526 {
          tunnel: w528 -> [_ w530]
          tunnel: [_ w529] -> w527
          frame False {
          }
          frame True {
            n268 = Increment(x=w530) -> (x+1=w531:i32)
            n269 = Number To Decimal String(number=w531) -> (decimal integer string=w532:string)  [unwired: 1 in]
            n270 = Concatenate Strings("Sched", w532) -> (w529:string)
          }
        }
      }
      n271 = property on="Close" class="Bool (strict)"("Value"=FALSE ("Close")) -> ()  [unwired: 2 in, 2 out]
      n272 = property on="Load" class="Bool (strict)"("Value"=TRUE ("Load")) -> ()  [unwired: 2 in, 2 out]
    }
    event "stop": Value Change {
      n273 = event-data() -> ()  [unwired: 1 in, 6 out]
      n274 = property on="Close" class="Bool (strict)"("Value"=TRUE ("Close")) -> ()  [unwired: 2 in, 2 out]
      n275 = property on="Load" class="Bool (strict)"("Value"=FALSE ("Load")) -> ()  [unwired: 2 in, 2 out]
    }
  }
  n276 = property on="selected sched" class="Str"("Value"=w4) -> ()  [unwired: 2 in, 2 out]
